vi "FP_TDMS_export_tool.vi"() -> ()   [LabVIEW 2018]
doc: "Tool for exporting TDMS files into CSV format."
uses:
  <vilib>/Utility/miscctls.llb/LVPointTypeDef.ctl
  <vilib>/Platform/TimedLoop/XDataNode/timing_clust.ctl
  <vilib>/Platform/TimedLoop/XDataNode/nitl_modes.ctl
  <vilib>/Platform/TimedLoop/XDataNode/wakeup.ctl
  <vilib>/Utility/sysdir.llb/System Directory Type.ctl
  <vilib>/Platform/TimedLoop/scheduler/LVUserAPI/_suppVIs/Create_1kHz_TSource.vi
  <vilib>/Utility/file.llb/Write Delimited Spreadsheet (string).vi
  <vilib>/platform/TimedLoop/XDataNode/XDataNode.xnode
  <vilib>/Platform/TimedLoop/XDataNode/XDNodeRunTimeDep.lvlib
panel:
  out "Progress bar":u8(slide) scale=0.0..100.0
  out "error out":errorcluster
  out "Files converted":u32
  out "Settings":bool[](array[boolean])
  out "Data":bool[](array[boolean])
  out "Errors array":string[](array[string])
  in  "Convert":bool
  out "Files to convert":u32
  out "Filelist":path[](array[path])
  in  "Open Folder":bool caption="Open File"
  in  "Stop":bool
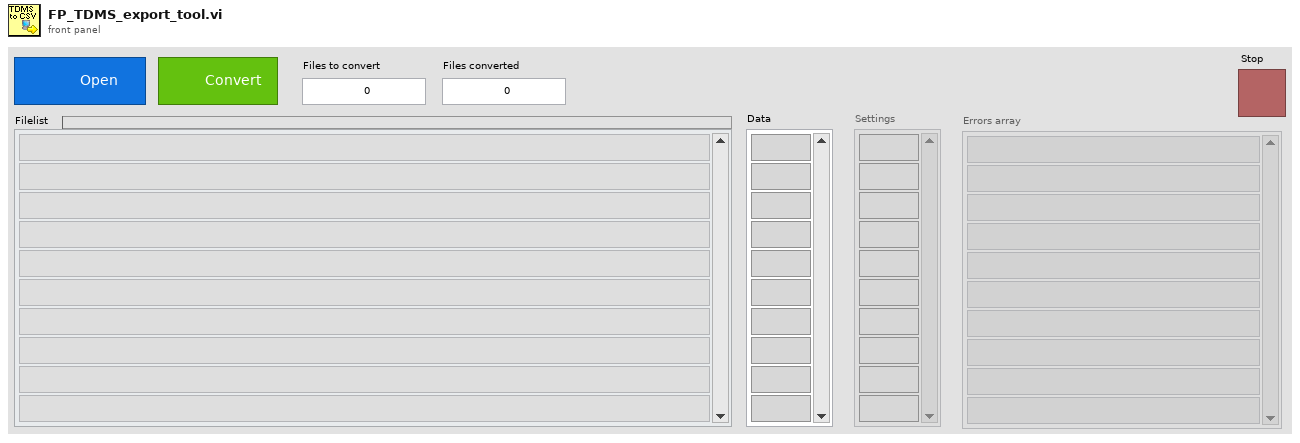
[diagram p1: front panel]
types:
  T1 = enum8{"Enabled", "Disabled", "Disabled and Grayed Out"}
  T2 = typedef "LVPointTypeDef.ctl" = cluster{"Horizontal":i16, "Vertical":i16}
  T3 = typedef "XDNodeRunTimeDep.lvlib/timing_clust.ctl" = cluster{"Expected End [f-1]":u64, "Actual End [f-1]":u64, "Finished Late? [f-1]":bool, "Expected End [i-1]":u64, "Actual End [i-1]":u64, "Finished Late? [i-1]":bool, "Expected Start [i]":u64, "Actual Start [i]":u64, "Expected Start [f]":u64, "Actual Start [f]":u64, "Source Name":string, "Structure Name":string, "Period":i64, "Deadline":i64, "Offset":i64, "Start":i64, "Priority":i32, "Timeout":i32, "Mode":T4, "Wakeup Reason":T5, "Error":errorcluster, "Source Type":string, "Secondary Source Type":string, "Global End Time":u64, "Global Start Time":u64, "Frame Duration":u64, "Iteration Duration":u64, "Assigned CPU":i32, "I/O Scan Engine Mode":u32}
  T4 = typedef "XDNodeRunTimeDep.lvlib/nitl_modes.ctl" = enum32{"No Change", "Process missed periods, maintain original phase", "Discard missed periods, maintain original phase", "Process missed periods, ignore original phase", "Discard missed periods, ignore original phase"}
  T5 = typedef "XDNodeRunTimeDep.lvlib/wakeup.ctl" = enum32{"Normal", "Aborted", "Asynchronous wakeup", "Timing source error", "Timed loop error", "Timeout"}
  T6 = enum32{"invalid app kind", "Development System", "Run Time System", "Student Edition", "Embedded LabVIEW", "Evaluation", "Custom"}
  T7 = typedef "System Directory Type.ctl" = i32
  T8 = cluster{"Raw coordinates data":dbl[][], "Absolute timestamp":string[], "Relative timestamp":string[], "Coordinates and speed":dbl[][], "Current zone and TTLs":u8[][], "Zones preference":string[], "Frame OK":u8[], "Stimulus presets array":cluster{"Event type":u16, "Time, s":sgl, "Stimulus, s":sgl, "Set/Clear":bool, "TTL out":u16, "Stim. has been set":bool}[], "Acquisition settings cluster out":cluster{"Researcher name":string, "N segments MIDFIELD":u8, "N segments BORDER":u8, "Radius, mm CENTER":u16, "Radius, mm MIDFIELD":u16, "Starting angle MIDFIELD":i16, "Starting angle BORDER":i16, "Cage diameter, mm":u16, "Bridge swap":bool, "Bridge V. offset":sgl, "Twisted neck":bool, "Offset H.":sgl, "Name prefix":string, "Stop at":dbl, "\"Stop at\" enabled":bool, "Settings loaded OK":bool}}
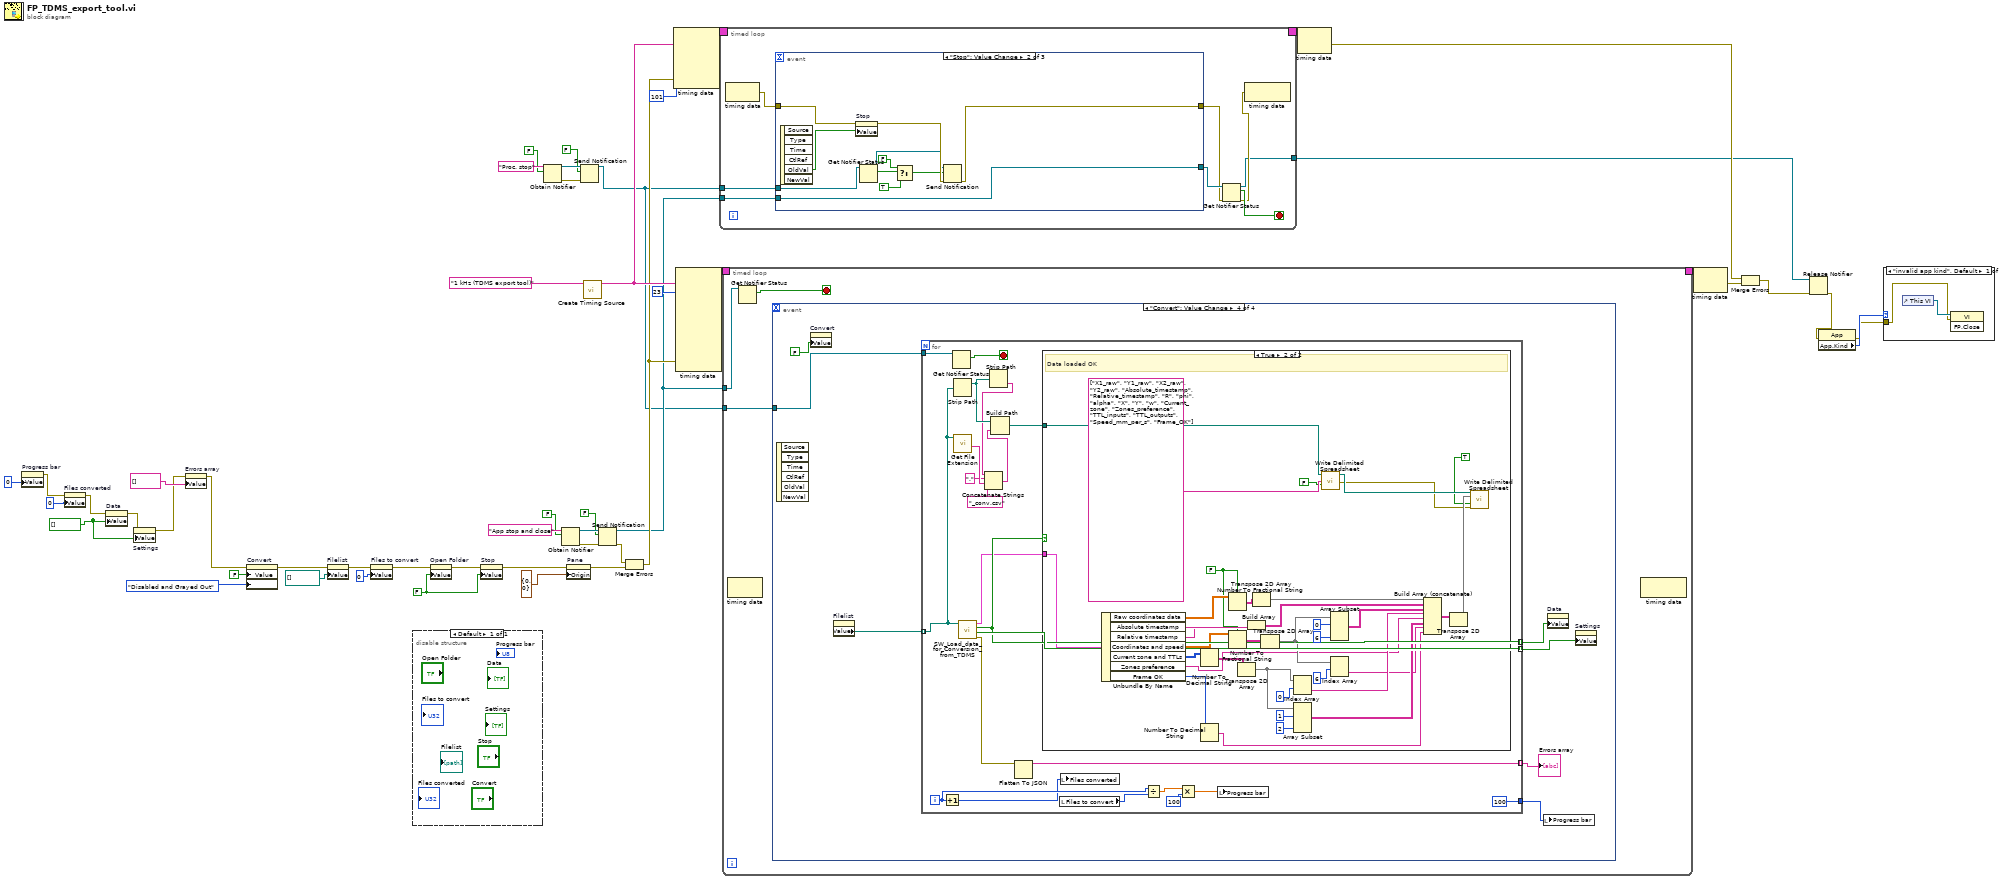
[diagram p0: block diagram]
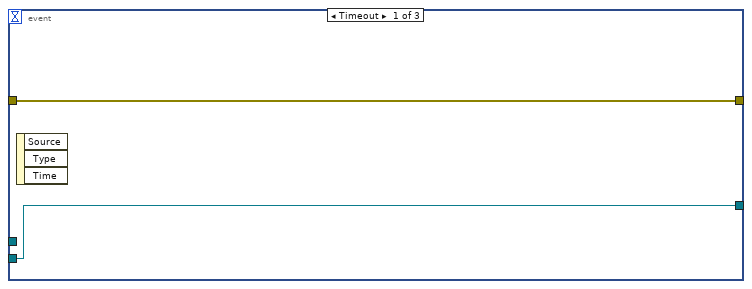
[diagram p3: hidden frame]
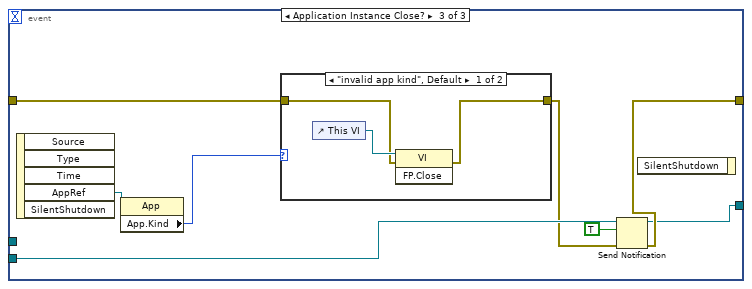
[diagram p4: hidden frame]
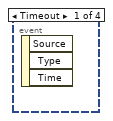
[diagram p6: hidden frame]
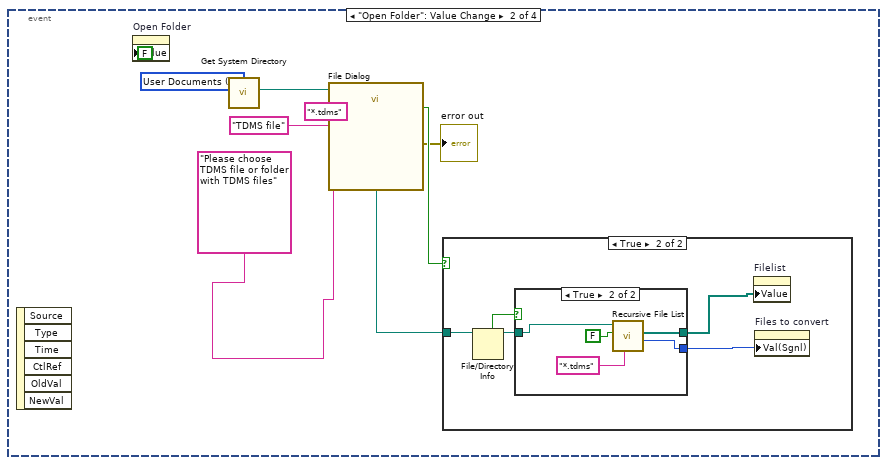
[diagram p7: hidden frame]
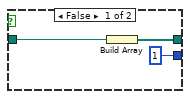
[diagram p9: hidden frame]
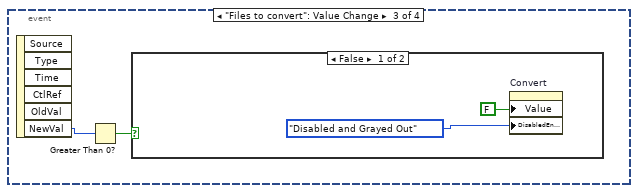
[diagram p10: hidden frame]
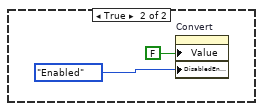
[diagram p11: hidden frame]
diagram:
  w33 = bool[] [] ("Array")
  w43 = FALSE ("Stop")
  n1 = property on="Progress bar" class="Slide (strict)"("Value"=u8 0 ("Progress bar")) -> (error out=w1:errorcluster)  [unwired: 2 in, 1 out]
  n2 = property on="Files converted" class="DigNum (strict)"(error in=w1, "Value"=u32 0 ("Files to converted")) -> (error out=w30:errorcluster)  [unwired: 1 in, 1 out]
  n3 = property on="Data" class="Arr"(error in=w30, "Value"=w33) -> (error out=w32:errorcluster)  [unwired: 1 in, 1 out]
  n4 = property on="Settings" class="Arr"(error in=w32, "Value"=w33) -> (error out=w31:errorcluster)  [unwired: 1 in, 1 out]
  n5 = property on="Errors array" class="Arr (strict)"(error in=w31, "Value"=string[] []) -> (error out=w35:errorcluster)  [unwired: 1 in, 1 out]
  n6 = property on="Convert" class="Bool (strict)"(error in=w35, "Value"=FALSE ("Convert"), "DisabledEnum"=T1."Disabled and Grayed Out" ("Disabled")) -> (error out=w38:errorcluster)  [unwired: 1 in, 1 out]
  n7 = property on="Filelist" class="Arr (strict)"(error in=w38, "Value"=path[] [] ("Files to process")) -> (error out=w39:errorcluster)  [unwired: 1 in, 1 out]
  n8 = property on="Files to convert" class="DigNum (strict)"(error in=w39, "Value"=u32 0 ("Number of files")) -> (error out=w42:errorcluster)  [unwired: 1 in, 1 out]
  n9 = disable-structure shown="Default" {
    frame Enabled {
    }
  }
  n10 = property on="Open Folder" class="Bool (strict)"(error in=w42, "Value"=w43) -> (error out=w44:errorcluster)  [unwired: 1 in, 1 out]
  n11 = property on="Stop" class="Bool (strict)"(error in=w44, "Value"=w43) -> (error out=w45:errorcluster)  [unwired: 1 in, 1 out]
  n12 = Obtain Notifier(name (unnamed)="Proc. stop", notification data type=FALSE) -> (notifier out=w6:refnum<notifier>, error out=w5:errorcluster)  [unwired: 2 in, 1 out]
  n13 = Obtain Notifier(name (unnamed)="App stop and close", notification data type=FALSE) -> (notifier out=w20:refnum<notifier>, error out=w19:errorcluster)  [unwired: 2 in, 1 out]
  n14 = property on="Pane" class="Pane"(error in=w45, "Origin"=T2 {"Horizontal"=0, "Vertical"=0}) -> (error out=w23:errorcluster)  [unwired: 1 in, 1 out]
  n15 = Send Notification(notification=FALSE, notifier=w6, error in (no error)=w5) -> (notifier out=w3:refnum<notifier>)  [unwired: 1 out]
  n16 = call-poly <vilib>:"Create Timing Source.vi"("name (in)"="1 kHz (TDMS export tool)") -> ("name (out)"=w25:string)  [unwired: 9 in, 1 out]
  n17 = Send Notification(notification=FALSE, notifier=w20, error in (no error)=w19) -> (notifier out=w15:refnum<notifier>, error out=w17:errorcluster)
  n18 = Merge Errors(w17, w23) -> (w18:errorcluster)
  n19 = node-c288(w25, i64 101 ("Period"), w18) -> (w27:T3)  [unwired: 2 in]
  n20 = node-c288(w25, i64 23 ("Period"), w18) -> (w50:T3)  [unwired: 7 in]
  n21 = timed-loop {
    timing: w27 -> [_]
    timing-out: [_] -> w26
    tunnel: w15 -> [w57]
    tunnel: [w52] -> w13
    tunnel: w3 -> [w51]
    stop <- w55 stop-if-true
    n22 = node-c288() -> (w58:errorcluster)  [unwired: 1 in]
    n23 = event shown="[1] \"Stop\": Value Change" {
      selector: _ -> [_ _ _]
      dyn-events: _ -> [_ _ _]
      timeout: _ -> [_ _ _]
      tunnel: w58 -> [w60 w71 w77]
      tunnel: [w60 w69 w74] -> w54
      tunnel: w57 -> [w59 w68 w76]
      tunnel: [w59 w68 w73] -> w56
      tunnel: w51 -> [_ w66 _]
      event Timeout {
        n24 = event-data() -> ()  [unwired: 1 in, 3 out]
      }
      event "Stop": Value Change {
        n25 = event-data() -> ("OldVal"=w67:bool)  [unwired: 1 in, 5 out]
        n26 = property on="Stop" class="Bool (strict)"(error in=w71, "Value"=w67) -> (error out=w70:errorcluster)  [unwired: 1 in, 1 out]
        n27 = Get Notifier Status(notifier=w66) -> (notifier out=w62:refnum<notifier>, current notification=w65:bool)  [unwired: 1 in, 3 out]
        n28 = Select(t=FALSE ("notification"), s=w65, f=TRUE) -> (s? t:f=w63:bool)
        n29 = Send Notification(notification=w63, notifier=w62, error in (no error)=w70) -> (error out=w69:errorcluster)  [unwired: 1 out]
      }
      event Application Instance Close? {
        n30 = event-data() -> ("AppRef"=w78:refnum<vi>)  [unwired: 1 in, 4 out]
        n31 = property class="App"(reference=w78) -> ("App.Kind"=w79:T6)  [unwired: 1 in, 2 out]
        n32 = case shown="\"invalid app kind\", Default" w79 {
          tunnel: w77 -> [w81 w83]
          tunnel: [w80 w83] -> w75
          frame "invalid app kind", Default {
            n33 = control-ref of="This VI"() -> (w82:refnum<vi>)
            n34 = invoke class="VI" method="FP.Close"(reference=w82, error in=w81) -> (error out=w80:errorcluster)  [unwired: 1 in, 2 out]
          }
          frame "Development System" {
          }
        }
        n35 = Send Notification(notification=TRUE, notifier=w76, error in (no error)=w75) -> (notifier out=w73:refnum<notifier>, error out=w74:errorcluster)
        n36 = event-data() -> ()  [unwired: 2 in, 1 out]
      }
    }
    n37 = Get Notifier Status(notifier=w56, error in (no error)=w54) -> (notifier out=w52:refnum<notifier>, current notification=w55:bool, error out=w53:errorcluster)  [unwired: 2 out]
    n38 = node-c288(w53) -> ()  [unwired: 1 out]
  }
  n39 = timed-loop {
    timing: w50 -> [_]
    timing-out: [_] -> w49
    tunnel: w15 -> [w91]
    tunnel: w3 -> [w89]
    stop <- w90 stop-if-true
    n40 = node-c288() -> ()  [unwired: 1 in, 1 out]
    n41 = Get Notifier Status(notifier=w91) -> (current notification=w90:bool)  [unwired: 1 in, 4 out]
    n42 = event shown="[3] \"Convert\": Value Change" {
      selector: _ -> [_ _ _ _]
      dyn-events: _ -> [_ _ _ _]
      timeout: _ -> [_ _ _ _]
      tunnel: w89 -> [_ _ _ w121]
      event Timeout {
        n43 = event-data() -> ()  [unwired: 1 in, 3 out]
      }
      event "Open Folder": Value Change {
        w96 = T7 2 items=["User Home"=0, "User Desktop"=1, "User Documents"=2, "User Application Data"=3, "User Preferences"=4, "User Temporary"=5, "Public Documents"=6, "Public Application Data"=7, "Public Preferences"=8, "Public Cache"=13, "System Core Libraries"=9, "System Installed Libraries"=10, "Application Files"=11, "Boot Volume Root"=12] ("system directory type")
        n44 = event-data() -> ()  [unwired: 1 in, 6 out]
        n45 = property on="Open Folder" class="Bool (strict)"("Value"=FALSE ("Open Folder")) -> ()  [unwired: 2 in, 2 out]
        n46 = call <vilib>:"Get System Directory.vi"("system directory type"=w96) -> ("system directory"=w95:path)  [unwired: 10 in]
        n47 = call "File Dialog"("start path"=w95, "prompt"="Please choose TDMS file or folder with TDMS files", "pattern (all files)"="*.tdms", "pattern label"="TDMS file") -> ("selected path"=w93:path, "exists"=w94:bool, "error out"=→"error out":errorcluster)  [unwired: 8 in, 1 out]
        n48 = case shown="True" w94 {
          tunnel: w93 -> [_ w105]
          frame False {
          }
          frame True {
            n49 = File/Directory Info(path=w105) -> (path out=w103:path, directory=w104:bool)  [unwired: 1 in, 5 out]
            n50 = case shown="True" w104 {
              tunnel: [w107 w110] -> w101
              tunnel: w103 -> [w108 w113]
              tunnel: [u32 1 ("Number of Files") w109] -> w102
              frame False {
                n51 = Build Array(w108) -> (w107:path[])
              }
              frame True {
                n52 = call <vilib>:"Recursive File List.vi"("pattern"="*.tdms", "Treat LLBs as Folders?"=FALSE, "Folder Path"=w113) -> ("Number of Files"=w109:i32, "All Files in Dir"=w110:path[])  [unwired: 4 in, 3 out]
              }
            }
            n53 = property on="Filelist" class="Arr (strict)"("Value"=w101) -> ()  [unwired: 2 in, 2 out]
            n54 = property on="Files to convert" class="DigNum (strict)"("Val(Sgnl)"=w102) -> ()  [unwired: 2 in, 2 out]
          }
        }
      }
      event "Files to convert": Value Change {
        n55 = event-data() -> ("NewVal"=w115:u32)  [unwired: 1 in, 5 out]
        n56 = Greater Than 0?(x=w115) -> (x > 0?=w114:bool)
        n57 = case shown="False" w114 {
          frame False {
            n58 = property on="Convert" class="Bool (strict)"("Value"=FALSE ("Convert"), "DisabledEnum"=T1."Disabled and Grayed Out" ("Disabled")) -> ()  [unwired: 2 in, 2 out]
          }
          frame True {
            n59 = property on="Convert" class="Bool (strict)"("Value"=FALSE ("Convert"), "DisabledEnum"=T1."Enabled" ("Disabled")) -> ()  [unwired: 2 in, 2 out]
          }
        }
      }
      event "Convert": Value Change {
        n60 = event-data() -> ()  [unwired: 1 in, 6 out]
        n61 = property on="Convert" class="Bool (strict)"("Value"=FALSE ("Convert")) -> ()  [unwired: 2 in, 2 out]
        n62 = property on="Filelist" class="Arr (strict)"() -> ("Value"=w125:path[])  [unwired: 2 in, 2 out]
        n63 = for {
          tunnel: w125 -> [w143] mode=indexing
          tunnel: [w148] -> w124 mode=indexing
          tunnel: [w145] -> w123 mode=indexing
          tunnel: [w146] -> w122 mode=indexing
          tunnel: w121 -> [w138]
          tunnel: [100] -> w120
          i -> [w132]
          stop <- w137 stop-if-true
          n64 = Increment(x=w132) -> (x+1=w130:i32)
          n65 = Get Notifier Status(notifier=w138) -> (current notification=w137:bool)  [unwired: 1 in, 4 out]
          n66 = Strip Path(path=w143) -> (stripped path=w129:path)  [unwired: 1 out]
          n67 = call <vilib>:"Get File Extension.vi"("file"=w143) -> ("filename without extension"=w142:string)  [unwired: 6 in, 4 out]
          n68 = call "SW_Load_data_for_Conversion_from_TDMS.vi"("Path to TDMS file"=w143) -> ("error out"=w147:errorcluster, "Settings loaded OK"=w146:bool, "Data loaded OK"=w145:bool, "Loaded data"=w144:T8)  [unwired: 4 in, 3 out]
          n69 = Strip Path(path=w129) -> (name=w128:string)  [unwired: 1 out]
          n70 = Concatenate Strings(w128, "." ("string"), w142, "_conv.csv" ("string")) -> (w140:string)
          n71 = Build Path(base path=w129, name or relative path=w140) -> (appended path=w139:path)
          n72 = Flatten To JSON(anything=w147) -> (JSON string=w148:string)  [unwired: 2 in, 1 out]
          n73 = case shown="True" w145 {
            tunnel: w144 -> [_ w183]
            tunnel: w139 -> [_ w181]
            frame False {
              # "Data is not loaded"
            }
            frame True {
              w168 = FALSE ("use system decimal point (T)")
              # "Data loaded OK"
              n74 = Unbundle By Name(w183) -> ("Raw coordinates data"=w180:dbl[][], "Absolute timestamp"=w178:string[], "Relative timestamp"=w177:string[], "Coordinates and speed"=w175:dbl[][], "Current zone and TTLs"=w172:u8[][], "Zones preference"=w159:string[], "Frame OK"=w170:u8[])
              n75 = Number To Decimal String(number=w172) -> (decimal integer string=w171:string[][])  [unwired: 1 in]
              n76 = Number To Decimal String(number=w170) -> (decimal integer string=w153:string[])  [unwired: 1 in]
              n77 = Number To Fractional String(use system decimal point (T)=w168, number=w180) -> (F-format string=w179:string[][])  [unwired: 2 in]
              n78 = Number To Fractional String(use system decimal point (T)=w168, number=w175) -> (F-format string=w167:string[][])  [unwired: 2 in]
              n79 = Transpose 2D Array(2D array=w171) -> (transposed array=w158:string[][])
              n80 = Build Array(w178, w177) -> (w174:string[][])
              n81 = Transpose 2D Array(2D array=w179) -> (transposed array=w173:string[][])
              n82 = Transpose 2D Array(2D array=w167) -> (transposed array=w165:string[][])
              n83 = Index Array(array=w158, index (row)=0) -> (element=w160:string[])  [unwired: 1 in]
              n84 = Array Subset(array=w158, index (row)=1 ("index"), length (row)=2 ("length")) -> (w155:string[][])  [unwired: 2 in]
              n85 = call-poly <vilib>:"Write Delimited Spreadsheet.vi"("file path (dialog if empty)"=w181, "1D data"=string[] ["X1_raw", "Y1_raw", "X2_raw", "Y2_raw", "Absolute_timestamp", "Relative_timestamp", "R", "phi", "alpha", "X", "Y", "w", "Current_zone", "Zones_preference", "TTL_inputs", "TTL_outputs", "Speed_mm_per_s", "Frame_OK"] ("appended array"), "append to file? (new file:F)"=FALSE) -> ("new file path (Not A Path if cancelled)"=w151:path, "error out"=w149:errorcluster)  [unwired: 11 in]
              n86 = Array Subset(array=w165, index (row)=0 ("index"), length (row)=6 ("length")) -> (w162:string[][])  [unwired: 2 in]
              n87 = Index Array(array=w165, index (row)=6) -> (element=w154:string[])  [unwired: 1 in]
              n88 = Build Array (concatenate)(w173, w174, w162, w160, w159, w155, w154, w153) -> (w176:string[][])
              n89 = Transpose 2D Array(2D array=w176) -> (transposed array=w169:string[][])
              n90 = call-poly <vilib>:"Write Delimited Spreadsheet.vi"("file path (dialog if empty)"=w151, "2D data"=w169, "append to file? (new file:F)"=TRUE, "error in (no error)"=w149) -> ()  [unwired: 10 in, 2 out]
            }
          }
          n91 = local read "Files to convert"() -> (w136:u32)
          n92 = local write "Files converted"(w130) -> ()
          n93 = Divide(x=w132, y=w136) -> (x/y=w135:dbl)
          n94 = Multiply(x=w135, y=100) -> (x*y=w133:dbl)
          n95 = local write "Progress bar"(w133) -> ()
        }
        "Errors array" <- w124
        n96 = local write "Progress bar"(w120) -> ()
        n97 = property on="Data" class="Arr"("Value"=w123) -> ()  [unwired: 2 in, 2 out]
        n98 = property on="Settings" class="Arr"("Value"=w122) -> ()  [unwired: 2 in, 2 out]
      }
    }
    n99 = node-c288() -> ()  [unwired: 1 in, 1 out]
  }
  n100 = node-c288(w26) -> (w14:errorcluster)
  n101 = node-c288(w49) -> (w28:errorcluster)
  n102 = Merge Errors(w14, w28) -> (w12:errorcluster)
  n103 = Release Notifier(notifier=w13, error in (no error)=w12) -> (error out=w10:errorcluster)  [unwired: 1 in, 2 out]
  n104 = property class="App"(error in=w10) -> (error out=w9:errorcluster, "App.Kind"=w11:T6)  [unwired: 1 in, 1 out]
  n105 = case shown="\"invalid app kind\", Default" w11 {
    tunnel: w9 -> [w186 _]
    frame "invalid app kind", Default {
      n106 = control-ref of="This VI"() -> (w187:refnum<vi>)
      n107 = invoke class="VI" method="FP.Close"(reference=w187, error in=w186) -> ()  [unwired: 1 in, 3 out]
    }
    frame "Development System" {
    }
  }
